vi "_Find Array of JSON Objects in JSON.vi"(7 "JSON Object Name":string, 8 "error in (no error)":errorcluster, 10 "JSON Array Name":string, 11 "JSON Config":string) -> (0 "error out":errorcluster, 3 "JSON Objects":string[](array[string]))   [LabVIEW 2021]
uses:
  <vilib>/JDP Science/JSONtext/Next JSON Value.vi
  <vilib>/JDP Science/JSONtext/String Subset.vi
  <vilib>/JDP Science/JSONtext/Parsing/Advance past next JSON Value (inlined COPY).vi
  <vilib>/JDP Science/JSONtext/Parsing/Advance past whitespace.vi
  <vilib>/JDP Science/JSONtext/Parsing/Advance past String.vi
  <vilib>/JDP Science/JSONtext/Parsing/Advance past Number.vi
  <vilib>/JDP Science/JSONtext/Parsing/Advance past Line Ending.vi
  <vilib>/JDP Science/JSONtext/Parsing/Parse Full Path or Item Name.vi
  <vilib>/JDP Science/JSONtext/Parsing/Advance past Array.vi
  <vilib>/JDP Science/JSONtext/Parsing/Advance past Object.vi
  <vilib>/JDP Science/JSONtext/support/Error Cluster From Code.vi
  <vilib>/JDP Science/JSONtext/Offset/Find Item Locations by Path.vi
  <vilib>/JDP Science/JSONtext/JSONtext.lvlib
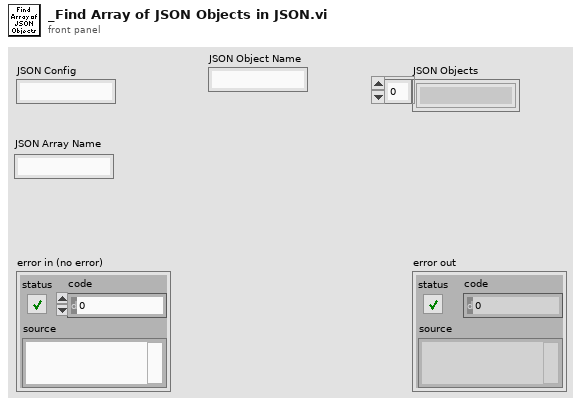
[diagram p1: front panel]
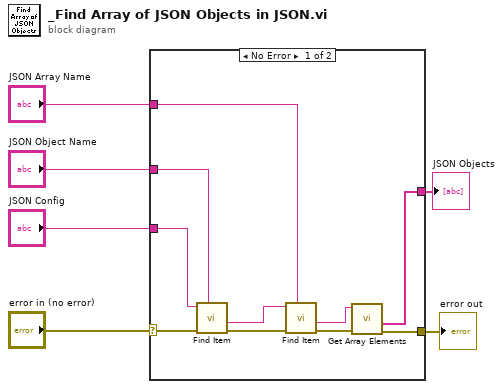
[diagram p0: block diagram]
diagram:
  n1 = case shown="No Error" "error in (no error)" {
    selector: "error in (no error)" -> [w13 w17]
    tunnel: [w16 _] -> w6
    tunnel: [w15 w17] -> w5
    tunnel: "JSON Object Name" -> [w14 _]
    tunnel: "JSON Config" -> [w12 _]
    tunnel: "JSON Array Name" -> [w7 _]
    frame No Error {
      n2 = call <vilib>:"Find Item.vi"("$Path or Item Name"=w14, "error in (no error)"=w13, "JSON"=w12) -> ("error out"=w10:errorcluster, "<JSON>"=w11:string)  [unwired: 5 in, 2 out]
      n3 = call <vilib>:"Find Item.vi"("$Path or Item Name"=w7, "error in (no error)"=w10, "JSON"=w11) -> ("error out"=w9:errorcluster, "<JSON>"=w8:string)  [unwired: 5 in, 2 out]
      n4 = call <vilib>:"Get Array Elements.vi"("error in (no error)"=w9, "JSON"=w8) -> ("error out"=w15:errorcluster, "<JSON>"=w16:string[])  [unwired: 7 in, 1 out]
    }
    frame Error {
    }
  }
  "JSON Objects" <- w6
  "error out" <- w5
